vi "testSendTelAndCmdFromClient.vi"(8 "error in (no error)":errorcluster) -> (0 "error out":errorcluster)   [LabVIEW 2018]
doc: "This VI sends commands from TCP client and receives the Ack from TCP server. Besides, TCP client sends telemetry to TCP server."
uses:
  <vilib>/addons/_JKI Toolkits/Caraya/classes/Assert/Assert Equal Value_Variant.vi
  src/TcpServer/TcpServer.lvclass
  <vilib>/addons/_JKI Toolkits/Caraya/classes/Test/Test.lvclass
  <vilib>/addons/_JKI Toolkits/Caraya/classes/Assert/Assert.lvclass
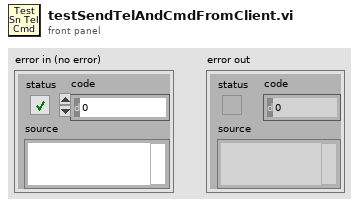
[diagram p1: front panel]
types:
  T1 = cluster{"CmdRead":refnum<user-event>, "EvtRead":refnum<user-event>, "GenRead":refnum<user-event>}
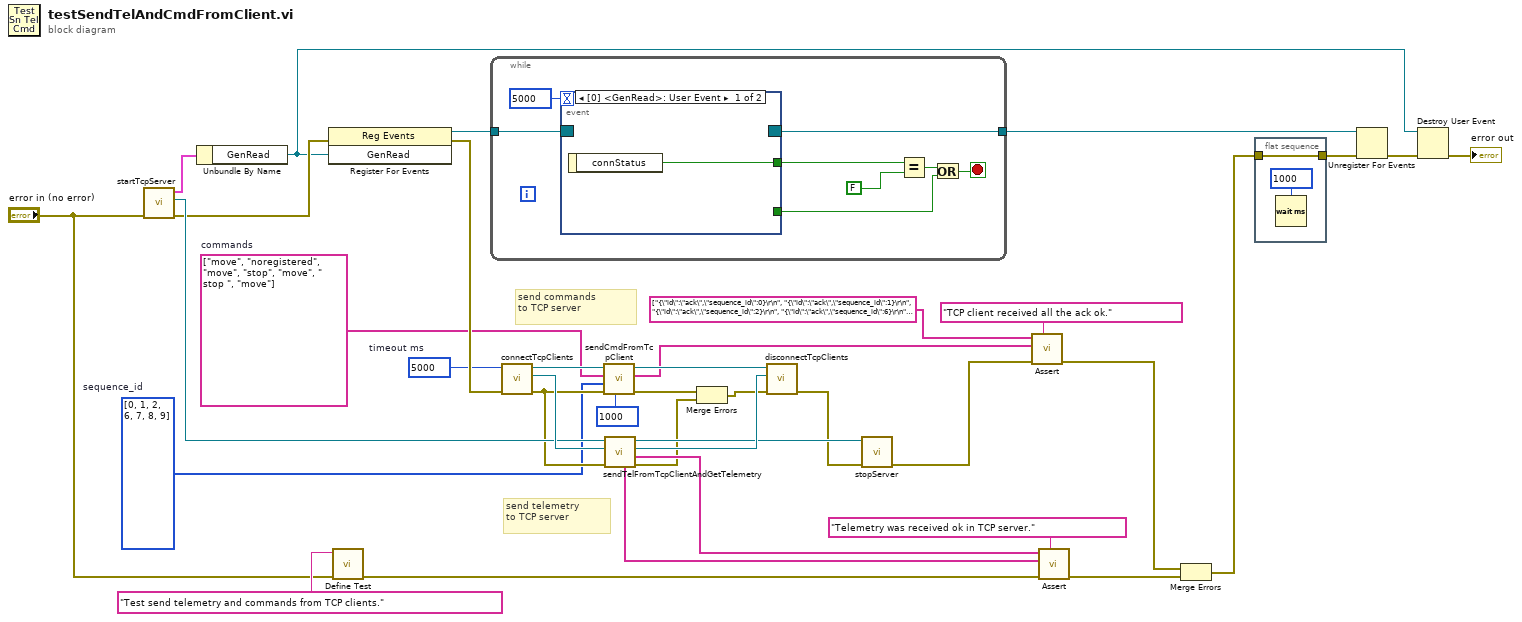
[diagram p0: block diagram]
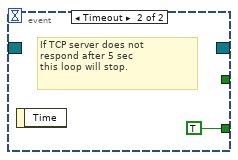
[diagram p2: hidden frame]
diagram:
  w4 = i32[] [0, 1, 2, 6, 7, 8, 9]  # sequence_id
  w5 = string[] ["move", "noregistered", "move", "stop", "move", " stop ", "move"]  # commands
  w6 = 5000  # timeout ms
  # "send telemetry\nto TCP server"
  # "send commands\nto TCP server"
  n1 = call "startTcpServer.vi"("error in (no error)"="error in (no error)") -> ("error out"=w8:errorcluster, "TcpServer out"=w21:refnum<class "TcpServer.lvclass">, "UserEvents"=w32:T1)  [unwired: 8 in]
  n2 = Unbundle By Name(w32) -> ("GenRead"=w1:refnum<user-event>)
  n3 = register-events(error in=w8, w1) -> (reference out=w37:refnum<event-registration>, error out=w7:errorcluster)  [unwired: 1 in]
  n4 = call <vilib>:"Define Test.vi"("error in (no error)"="error in (no error)", "Label (VI Title)"="Test send telemetry and commands from TCP clients.") -> ("error out"=w29:errorcluster)  [unwired: 9 in]
  n5 = while {
    tunnel: w37 -> [w45]
    tunnel: [w44] -> w36
    stop <- w42 stop-if-true
    n6 = event shown="[0] <GenRead>: User Event" {
      selector: w45 -> [_ _]
      dyn-events: [_ _] -> w44
      timeout: 5000 -> [_ _]
      tunnel: [w46 _] -> w43
      tunnel: [_ TRUE] -> w39
      event User Event {
        n7 = event-data() -> ("connStatus"=w46:bool)  [unwired: 1 in]
      }
      event Timeout {
        # "If TCP server does not\nrespond after 5 sec\nthis loop will stop."
        n8 = event-data() -> ()  [unwired: 1 in, 1 out]
      }
    }
    n9 = Equal?(x=w43, y=FALSE) -> (x = y?=w40:bool)
    n10 = Or(x=w40, y=w39) -> (x .or. y?=w42:bool)
  }
  n11 = call "connectTcpClients.vi"("error in (no error)"=w7, "timeout ms"=w6) -> ("error out"=w10:errorcluster, "tel connection ID out"=w31:refnum<k5>, "cmd connection ID out"=w24:refnum<k5>)  [unwired: 7 in]
  n12 = call "sendCmdFromTcpClient.vi"("timeout ms (1000)"=1000, "error in (no error)"=w10, "sequence_id"=w4, "commands"=w5, "connectionID"=w24) -> ("error out"=w16:errorcluster, "ack received"=w11:string[], "connectionID"=w20:refnum<k5>)  [unwired: 4 in]
  n13 = call "sendTelFromTcpClientAndGetTelemetry.vi"("error in (no error)"=w10, "tel connection ID in"=w31, "TcpServer in"=w21) -> ("error out"=w14:errorcluster, "telemetry sent"=w27:string[], "tel connection ID out"=w19:refnum<k5>, "TcpServer out"=w18:refnum<class "TcpServer.lvclass">, "telemetry received"=w17:string[])  [unwired: 4 in]
  n14 = Merge Errors(w16, w14) -> (w15:errorcluster)
  n15 = call "disconnectTcpClients.vi"("error in (no error)"=w15, "tel connection ID in"=w19, "cmd connection ID in"=w20) -> ("error out"=w13:errorcluster)  [unwired: 8 in]
  n16 = call "stopServer.vi"("error in (no error)"=w13, "tcpServer in"=w18) -> ("error out"=w12:errorcluster)  [unwired: 8 in, 1 out]
  n17 = call-poly <vilib>:"Assert.vi"("Label"="TCP client received all the ack ok.", "error in (no error)"=w12, "Y"=w11, "X"=string[] ["{\"id\":\"ack\",\"sequence_id\":0}\r\n", "{\"id\":\"ack\",\"sequence_id\":1}\r\n", "{\"id\":\"ack\",\"sequence_id\":2}\r\n", "{\"id\":\"ack\",\"sequence_id\":6}\r\n", "{\"id\":\"noack\",\"sequence_id\":3}\r\n", "{\"id\":\"noack\",\"sequence_id\":4}\r\n", "{\"id\":\"noack\",\"sequence_id\":5}\r\n", "{\"id\":\"ack\",\"sequence_id\":7}\r\n", "{\"id\":\"ack\",\"sequence_id\":8}\r\n", "{\"id\":\"ack\",\"sequence_id\":9}\r\n"] ("ack received")) -> ("error out"=w22:errorcluster)  [unwired: 7 in]
  n18 = call-poly <vilib>:"Assert.vi"("Label"="Telemetry was received ok in TCP server.", "error in (no error)"=w29, "Y"=w17, "X"=w27) -> ("error out"=w25:errorcluster)  [unwired: 7 in]
  n19 = Merge Errors(w22, w25) -> (w26:errorcluster)
  n20 = flat-sequence {
    tunnel: w26 -> [w48]
    tunnel: [w48] -> w34
    frame #0 {
      n21 = Wait (ms)(milliseconds to wait=u32 1000) -> ()  [unwired: 1 out]
    }
  }
  n22 = Unregister For Events(event registration refnum=w36, error in=w34) -> (error out=w35:errorcluster)
  n23 = Destroy User Event(user event=w1, error in=w35) -> (error out=→"error out":errorcluster)
